vi "Tank Drive.vi"() -> ()   [LabVIEW 2015]
doc: "Tank Drive Example\n\nThis example shows how to implement tank drive and uses two joysticks for input.\n\nThis example expects a USB cable connected from your development PC to the Type B USB Jack (next to the power input) on the roboRIO.\n\nThis example requires the Driver Station to be running with Teleoperated Enabled."
uses:
  <vilib>/Rock Robotics/SystemInterfaces/DIO/FPGA_DIOPWMChannel.ctl
  <vilib>/Rock Robotics/WPI/Joystick/WPI_JoystickDeviceEnum.ctl
  <vilib>/Rock Robotics/WPI/RobotDrive/WPI_RobotDriveOpen2MotorWithTalon.vi
  <vilib>/Rock Robotics/WPI/RobotDrive/WPI_RobotDriveArcadeDrive_Standard(NoSaturation).vi
panel:
  out "Numeric":dbl
  in  "LeftStick":T1
  in  "Left Motor (PWM channel)":T2
  in  "Right Motor (PWM channel)":T2=enum."PWM 1"
  in  "stop":bool
  # "Set these inputs before running."
  # "This example requires the Driver Station to be running with Teleoperated Enabled."
  # "PWM cables"
  # "This shows wiring for Talon speed controllers.  The wiring is similar for Victor and Jaguar controllers.  If you change the controller type, you must also select the appropriate instance of the Motor Open VI on the diagram."
  # "Power\nTerminals"
  # "Motor\nTerminals"
  # "+"
  # "+"
  # "M"
  # "B"
  # "Power\nTerminals"
  # "Motor\nTerminals"
  # "+"
  # "+"
  # "M"
  # "B"
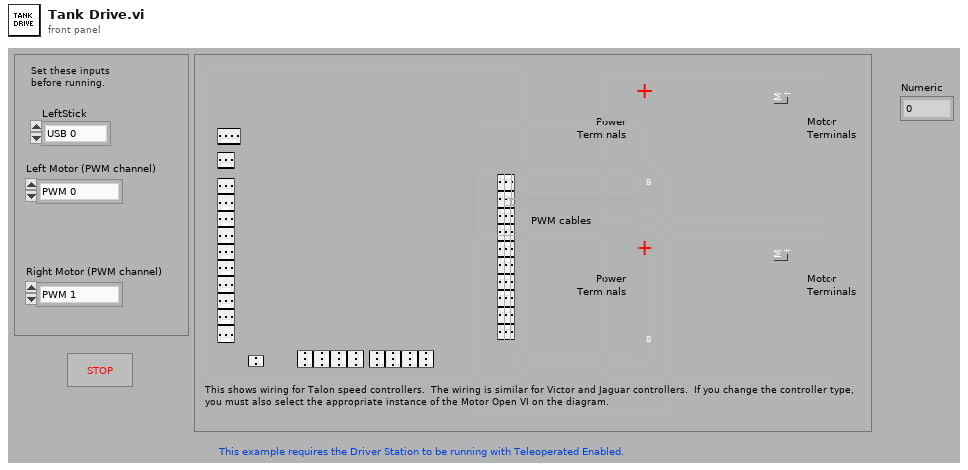
[diagram p1: front panel]
types:
  T1 = typedef "WPI_JoystickDeviceEnum.ctl" = enum16{"USB 0", "USB 1", "USB 2", "USB 3", "USB 4", "USB 5"}
  T2 = typedef "FPGA_DIOPWMChannel.ctl" = enum8{"PWM 0", "PWM 1", "PWM 2", "PWM 3", "PWM 4", "PWM 5", "PWM 6", "PWM 7", "PWM 8", "PWM 9", "PWM MXP 0", "PWM MXP 1", "PWM MXP 2", "PWM MXP 3", "PWM MXP 4", "PWM MXP 5", "PWM MXP 6", "PWM MXP 7", "PWM MXP 8", "PWM MXP 9", "Invalid"}
  T3 = typedef "WPI_JoystickDevRef.ctl" = cluster{"Device":T1}
  T4 = typedef "WPI_RobotDriveDevRef.ctl" = cluster{"DevStatus":errorcluster, "Motors[]":T5[], "Square Inputs":bool, "Max Output":dbl}
  T5 = typedef "WPI_MotorControlDeviceRef.ctl" = cluster{"DeviceStatus":errorcluster, "Type":T6, "PWM":cluster{"PWM Channel":T2, "DeadBand":T7}, "CAN":cluster{"Device Number":u8, "Control Mode":T8, "Semaphore":T9, "Max Vout":dbl, "TalonSRX Control Mode":T10}, "Invert":bool}
  T6 = typedef "WPI_MotorControlType.ctl" = enum16{"PWM", "CAN", "CANTalonSRX"}
  T7 = typedef "WPI_PWMDeadband.ctl" = cluster{"Name":string, "maxPositivePwm":i32, "minPositivePwm":i32, "centerPwm":i32, "maxNegativePwm":i32, "minNegativePwm":i32, "angularRange":u16}
  T8 = typedef "WPI_CANJaguar_ControlMode.ctl" = enum8{"Percent VBus", "Current", "Speed", "Position", "Voltage"}
  T9 = typedef "Semaphore RefNum" = refnum<k1>
  T10 = typedef "WPI_CANTalonSRX_APIControlMode.ctl" = enum8{"Percent VBus", "Speed", "Position", "Slave", "Unchanged / Invalid", "Voltage Compensation", "Current", "Motion Profile"}
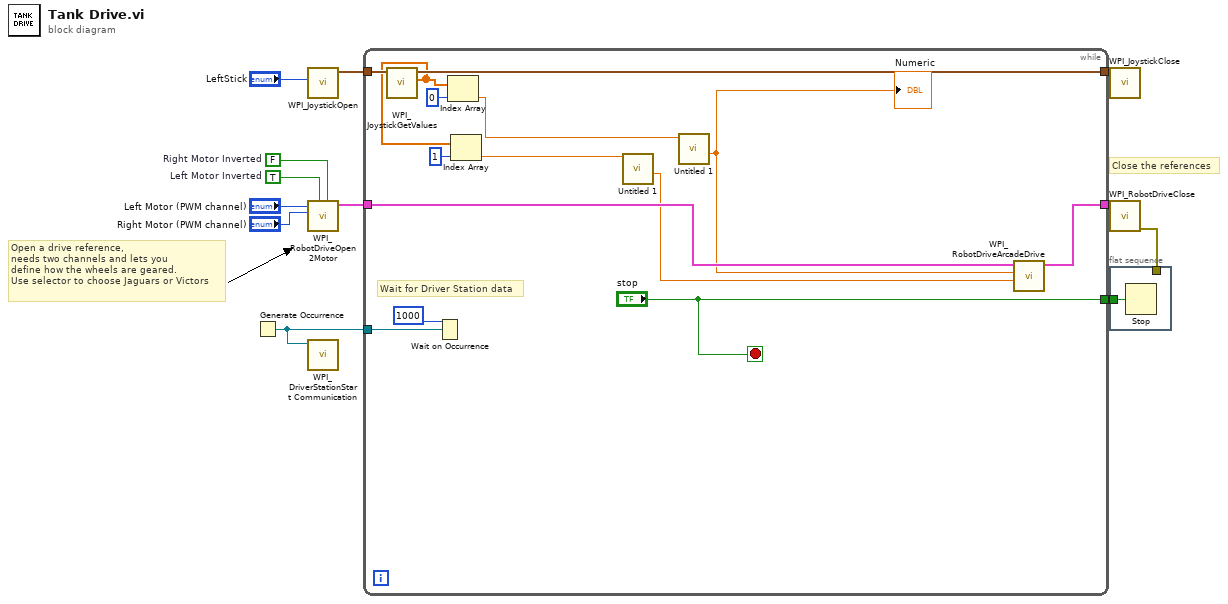
[diagram p0: block diagram]
diagram:
  w6 = FALSE  # Right Motor Inverted
  w7 = TRUE  # Left Motor Inverted
  # "Close the references"
  # "Open a drive reference,\nneeds two channels and lets you\ndefine how the wheels are geared.\nUse selector to choose Jaguars or Victors"
  n1 = Generate Occurrence() -> (w8:refnum<k4>)
  n2 = call <vilib>:"WPI_JoystickOpen.vi"("JoystickDevice"="LeftStick") -> ("JoystickDevRef"=w4:T3)  [unwired: 10 out]
  n3 = call-poly <vilib>:"WPI_RobotDriveOpen2Motor.vi"("Right Motor Inverted"=w6, "Left Motor Inverted"=w7, "Right Motor"="Right Motor (PWM channel)", "Left Motor"="Left Motor (PWM channel)") -> ("RobotDriveDevRef"=w10:T4)  [unwired: 1 in, 6 out]
  n4 = call <vilib>:"WPI_DriverStationStart Communication.vi"("occurrence"=w8) -> ()  [unwired: 1 in, 10 out]
  n5 = while {
    tunnel: w10 -> [w21]
    tunnel: [w22] -> w9
    tunnel: w8 -> [w26]
    tunnel: ["stop"] -> w2
    tunnel: w4 -> [w23]
    tunnel: [w20] -> w3
    stop <- "stop" stop-if-true
    # "Wait for Driver Station data"
    n6 = call <vilib>:"WPI_JoystickGetValues.vi"("JoystickDevRef"=w23) -> ("Axes"=w16:dbl[], "JoystickDevRef"=w20:T3)  [unwired: 6 in, 3 out]
    n7 = Wait on Occurrence(2:w26, 3:1000 ("ms timeout (-1)")) -> ()  [unwired: 2 out]
    n8 = Index Array(array=w16, index=0) -> (element=w18:dbl)
    n9 = Index Array(array=w16, index=1) -> (element=w14:dbl)
    n10 = call "Untitled 1.vi"("Numeric"=w14) -> ("s? t:f"=w13:dbl)  [unwired: 10 in]
    n11 = call "Untitled 1.vi"("Numeric"=w18) -> ("s? t:f"=w17:dbl)  [unwired: 10 in]
    "Numeric" <- w17
    n12 = call-poly <vilib>:"WPI_RobotDriveArcadeDrive.vi"("Y axis value"=w13, "X axis value"=w17, "RobotDriveDevRef"=w21) -> ("RobotDriveDevRef"=w22:T4)  [unwired: 6 in, 2 out]
  }
  n13 = call <vilib>:"WPI_JoystickClose.vi"("JoystickDevRef"=w3) -> ()  [unwired: 11 out]
  n14 = call <vilib>:"WPI_RobotDriveClose.vi"("RobotDriveDevRef"=w9) -> ("error out"=w1:errorcluster)  [unwired: 1 in, 9 out]
  n15 = flat-sequence {
    tunnel: w2 -> [w27]
    tunnel: w1 -> [_]
    frame #0 {
      n16 = Stop(stop? (T)=w27) -> ()
    }
  }
